vi "Convert PWM Module to Slot Configuration.vi"(8 "error in":errorcluster, 9 "module":refnum<class "Module.lvclass">, 10 "RSI module":refnum<class "RSI Module.lvclass">=refnum, 11 "slot ref in":T1 format="%.0x") -> (0 "error out":errorcluster, 3 "slot ref out":T1 format="%.0x")   [LabVIEW 2019, in "Scan Engine Scripting.lvlib"]
uses:
  Scan Engine Scripting.lvlib
  Modules.lvlibp/SD Module/SD Module.lvclass
  Modules/Module/Module.lvclass
  <vilib>/NI VeriStand/Custom Device API/Custom Device Item Ref.ctl
  <vilib>/NI VeriStand/Custom Device API/Custom Device API.lvlib
  Modules.lvlibp/RSI Module/RSI Module.lvclass
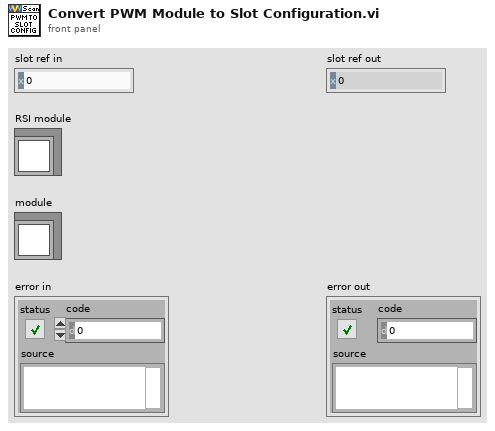
[diagram p1: front panel]
types:
  T1 = typedef "Custom Device API.lvlib/Custom Device Item Ref.ctl" = u64
  T2 = typedef "Scan Engine Scripting.lvlib/pwm channel settings.ctl" = cluster{"name":string, "default value":dbl, "frequency":T3}
  T3 = typedef "Scan Engine Scripting.lvlib/PWM Output Channel.lvclass/Frequency.ctl" = enum16{"1 Hz (1,000,000 us)", "50 Hz (20,000 us)", "250 Hz (4,000 us)", "500 Hz (2,000 us)", "1 kHz (1,000 us)", "5 kHz (200 us)", "10 kHz (100 us)", "20 kHz (50 us)"}
  T4 = typedef "Modules.lvlibp/SD Module.lvclass/PWM.ctl" = cluster{"PWM Channels":T5[]}
  T5 = typedef "Modules.lvlibp/SD Module.lvclass/PWM Channel.ctl" = cluster{"PWM frequency":u32}
  T6 = typedef "Modules.lvlibp/Custom Device API.lvlib/Custom Device Item Ref.ctl" = u64
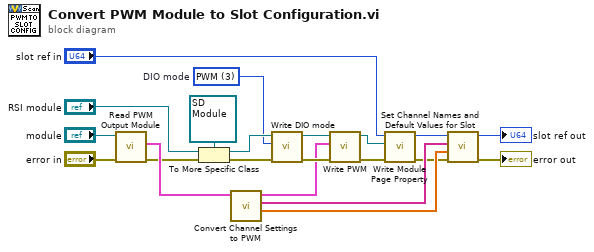
[diagram p0: block diagram]
diagram:
  w1 = u32 3 items=["Normal", "Counter", "Counter Slave", "PWM", "Quadrature"]  # DIO mode
  n1 = call-dynamic "Read PWM Output Module.vi"("error in"="error in", "module in"="module") -> ("error out"=w5:errorcluster, "channel settings"=w10:T2[])  [unwired: 7 in, 1 out]
  n2 = To More Specific Class(target class=refnum<class "SD Module.lvclass"> refnum ("Modules.lvlibp:SD Module.lvclass"), reference="RSI module", error in=w5) -> (specific class reference=w7:refnum<class "SD Module.lvclass">, error out=w9:errorcluster)
  n3 = call "Convert Channel Settings to PWM.vi"("channel settings"=w10) -> ("channel default values"=w16:dbl[], "channel names"=w15:string[], "PWM"=w11:T4)  [unwired: 8 in]
  n4 = call-dynamic "Write DIO mode.vi"("error in (no error)"=w9, "DIO mode"=w1, "SD Module in"=w7) -> ("error out"=w21:errorcluster, "SD Module out"=w20:refnum<class "SD Module.lvclass">)  [unwired: 7 in]
  n5 = call-dynamic "Write PWM.vi"("error in (no error)"=w21, "PWM"=w11, "SD Module in"=w20) -> ("error out"=w12:errorcluster, "SD Module out"=w19:refnum<class "SD Module.lvclass">)  [unwired: 7 in]
  n6 = call "Write Module Page Property.vi"("error in (no error)"=w12, "RSI Module"=w19, "Node Ptr In"="slot ref in") -> ("error out"=w13:errorcluster, "Node Ptr Out"=w14:T6)  [unwired: 6 in, 1 out]
  n7 = call "Set Channel Names and Default Values for Slot.vi"("error in"=w13, "default values"=w16, "channel names"=w15, "slot ref in"=w14) -> ("error out"=→"error out":errorcluster, "slot ref out"=→"slot ref out":T1)  [unwired: 6 in]
